vi "AFM_sync_volumetric_scan.vi"() -> ()   [LabVIEW 2017]
uses:
  <vilib>/DAQmx/write.llb/DAQmx Write (Analog DBL 1Chan 1Samp).vi
  <vilib>/DAQmx/write.llb/DAQmx Write (Analog 1D DBL NChan 1Samp).vi
  <vilib>/DAQmx/write.llb/DAQmx Write (Analog 2D DBL NChan NSamp).vi
  <vilib>/Utility/file.llb/Read Delimited Spreadsheet (DBL).vi
  <vilib>/DAQmx/create/channels.llb/DAQmx Create Channel (AO-Voltage-Basic).vi
  <vilib>/DAQmx/miscellaneous.llb/DAQmx Fill In Error Info.vi
  <vilib>/measure/mascope.llb/Transition Measurements 1 chan.vi
  <vilib>/DAQmx/configure/timing.llb/DAQmx Timing (Sample Clock).vi
  <vilib>/DAQmx/configure/trigger.llb/DAQmx Start Trigger (Digital Edge).vi
  <resource>/objmgr/daqmx.rc
  <vilib>/measure/NI_MAPro.lvlib
panel:
  out "Sampling rate":i32
  out "ETL3":waveform(dbl)(graph)
  out "mirror y":waveform(dbl)(graph)
  out "mirror x":waveform(dbl)(graph)
  out "561":waveform(dbl)(graph)
  out "488":waveform(dbl)(graph)
  out "camera":waveform(dbl)(graph)
  out "mirx transition duration":dbl
  out "transition duration":dbl
  out "etl3 timing array":dbl[](array[numeric])
  out "mirror y timing array":dbl[](array[numeric])
  out "mirror x timing array":dbl[](array[numeric])
  out "561 timing array":dbl[](array[numeric])
  out "488 timing array":dbl[](array[numeric])
  out "camera timing array":dbl[](array[numeric])
  out "etl raw":dbl[](array[numeric])
  out "miry raw":dbl[](array[numeric])
  out "mirx raw":dbl[](array[numeric])
  out "561 Intensity":dbl
  out "488 Intensity":dbl
  out "Off Time":dbl
  out "On Time":dbl
  out "Number of slices":dbl
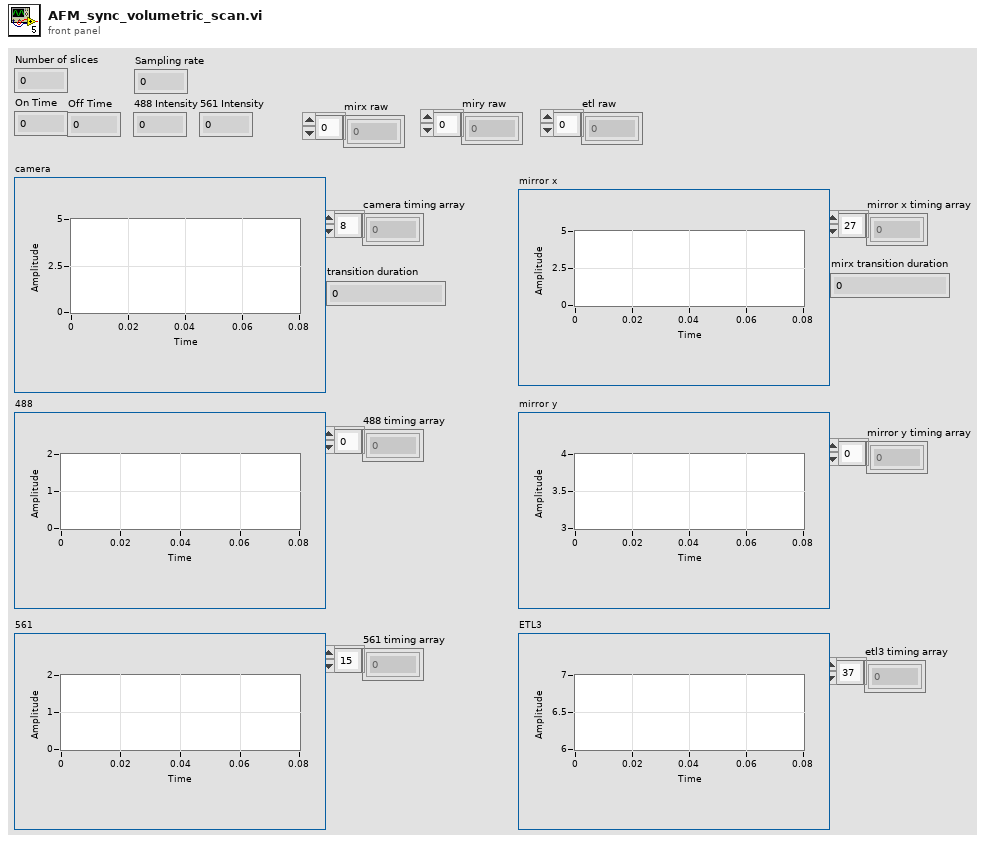
[diagram p1: front panel]
types:
  T1 = enum32{"Invalid", "Standard", "Closed", "Hidden", "Minimized", "Maximized"}
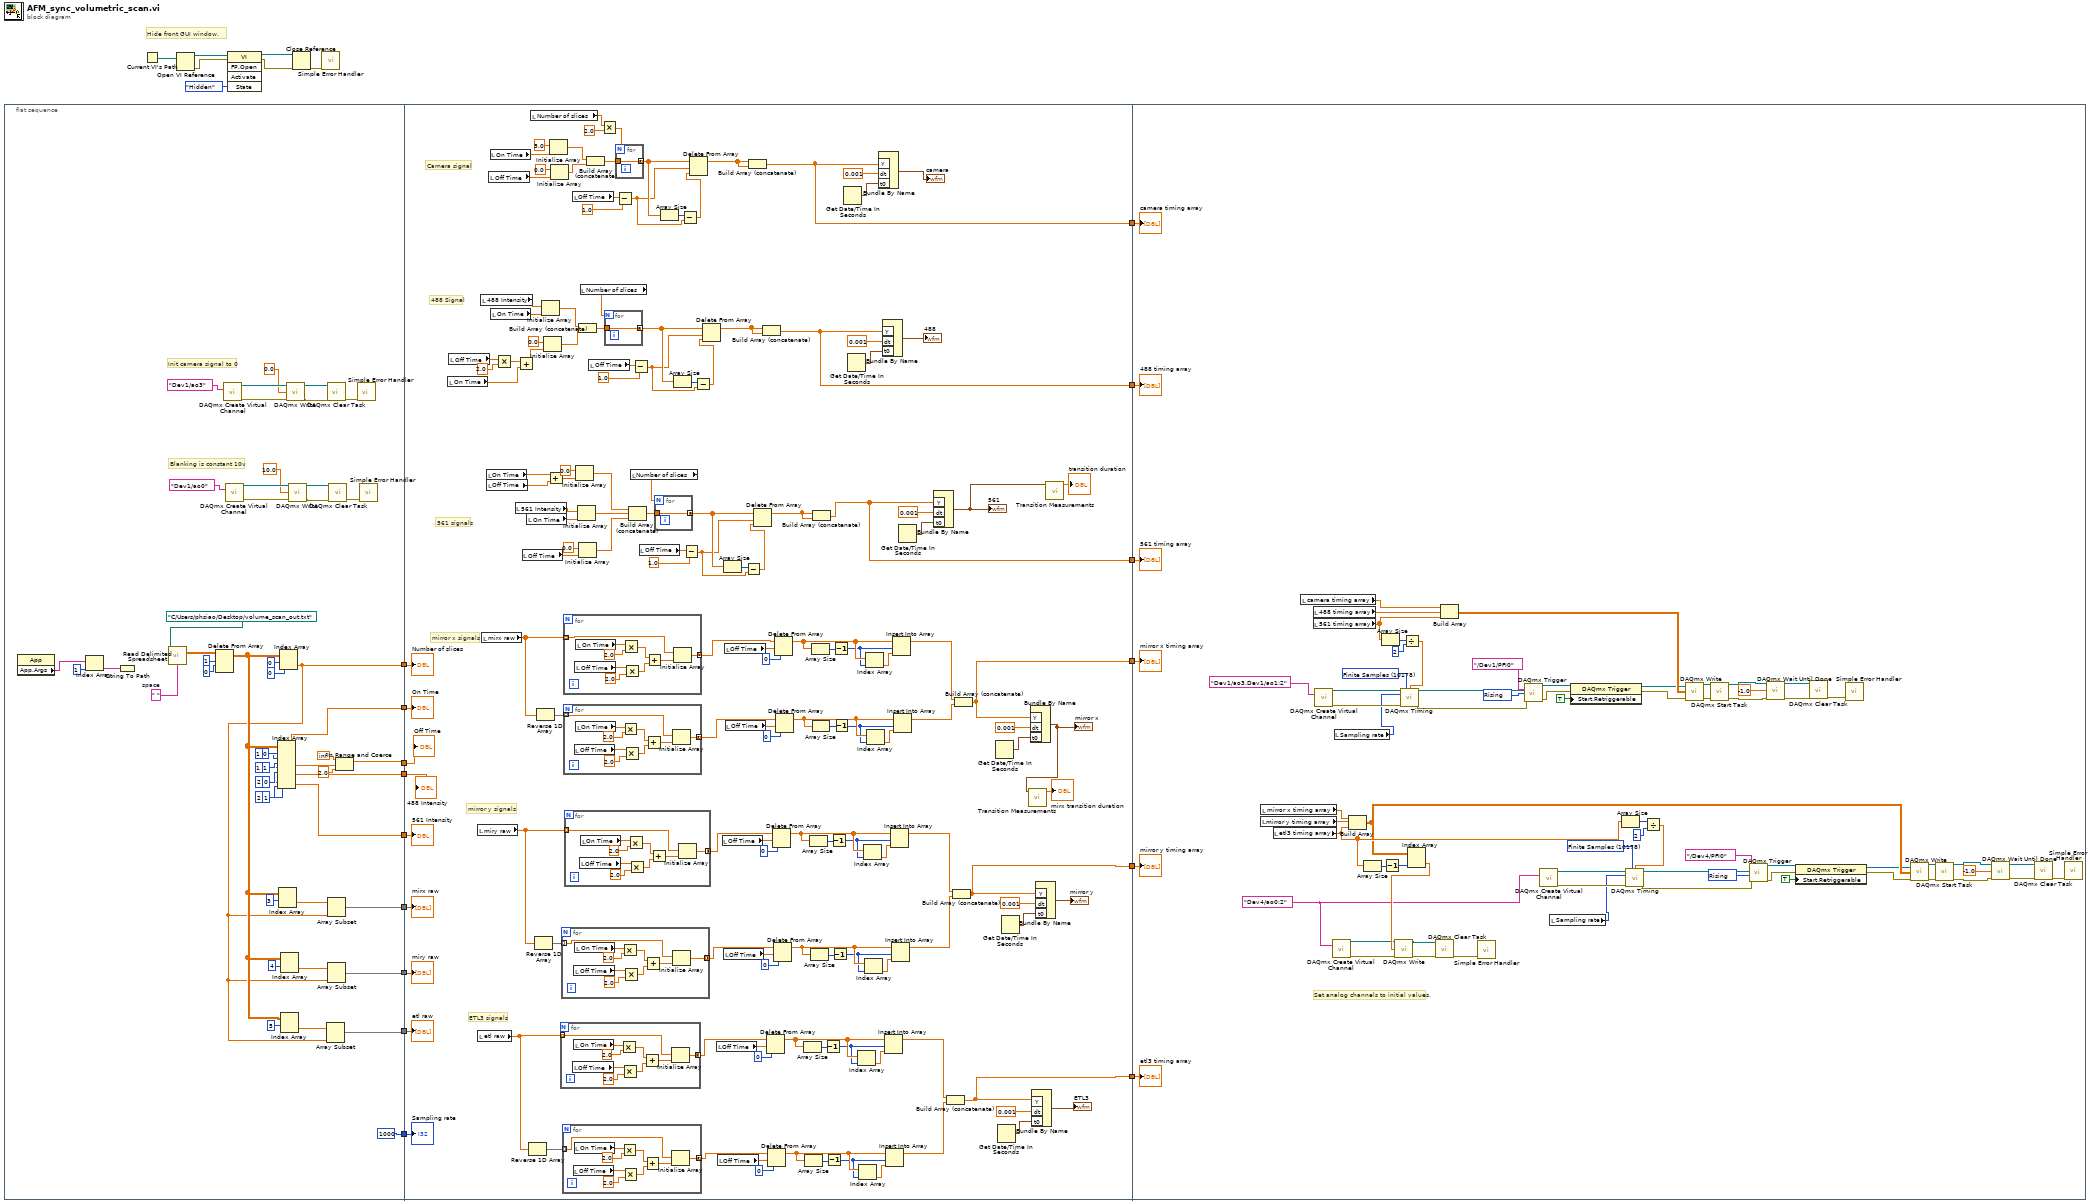
[diagram p0: block diagram]
diagram:
  # "Hide front GUI window."
  n1 = flat-sequence {
    tunnel: [w48] -> w22
    tunnel: [w47] -> w21
    tunnel: [w46] -> w20
    tunnel: [w45] -> w19
    tunnel: [w44] -> w18
    tunnel: [w43] -> w17
    tunnel: [w42] -> w16
    tunnel: [w41] -> w15
    tunnel: [1000] -> w8
    tunnel: w22 -> [w96]
    tunnel: w21 -> [w95]
    tunnel: w20 -> [w94]
    tunnel: w19 -> [w93]
    tunnel: w18 -> [w92]
    tunnel: w17 -> [w91]
    tunnel: w16 -> [w90]
    tunnel: w15 -> [w89]
    tunnel: [w88] -> w14
    tunnel: [w87] -> w13
    tunnel: [w86] -> w12
    tunnel: [w85] -> w11
    tunnel: [w84] -> w10
    tunnel: [w83] -> w9
    tunnel: w8 -> [w74]
    tunnel: w14 -> [w283]
    tunnel: w13 -> [w282]
    tunnel: w12 -> [w281]
    tunnel: w11 -> [w280]
    tunnel: w10 -> [w279]
    tunnel: w9 -> [w278]
    frame #0 {
      w49 = " "  # space
      # "Init camera signal to 0"
      # "Blanking is constant 10v"
      n2 = property class="App"() -> ("App.Args"=w24:string[])  [unwired: 2 in, 2 out]
      n3 = Index Array(array=w24, index=1) -> (element=w23:string)
      n4 = String To Path(string=w23) -> ()  [unwired: 1 out]
      n5 = call-poly <vilib>:"Read Delimited Spreadsheet.vi"("file path (dialog if empty)"=path "C:/Users/phsiao/Desktop/volume_scan_out.txt", "delimiter (\\t)"=w49) -> ("all rows"=w68:dbl[][])  [unwired: 8 in, 5 out]
      n6 = Delete From Array(array=w68, length=1, index (row)=0) -> (array with subset deleted=w69:dbl[][])  [unwired: 1 in, 1 out]
      n7 = call-poly <vilib>:"DAQmx Create Virtual Channel.vi"("physical channels"=tag "Dev1/ao3") -> ("task out"=w29:refnum<k21>, "error out"=w30:errorcluster)  [unwired: 13 in]
      n8 = call-poly <vilib>:"DAQmx Create Virtual Channel.vi"("physical channels"=tag "Dev1/ao0") -> ("task out"=w37:refnum<k21>, "error out"=w38:errorcluster)  [unwired: 13 in]
      n9 = Index Array(array=w69, index (row) #1=1 ("index (row)"), index (col) #1=0 ("disabled index (col)"), index (row) #2=1 ("index (row)"), index (col) #2=1 ("disabled index (col)"), index (row) #3=2 ("index (row)"), index (col) #3=0 ("disabled index (col)"), index (row) #4=2 ("index (row)"), index (col) #4=1 ("disabled index (col)")) -> (element #1=w47:dbl, element #2=w73:dbl, element #3=w45:dbl, element #4=w44:dbl)
      n10 = Index Array(array=w69, index (row)=3) -> (element=w70:dbl[])  [unwired: 1 in]
      n11 = Index Array(array=w69, index (row)=0, index (col)=0 ("disabled index (col)")) -> (element=w48:dbl)
      n12 = Index Array(array=w69, index (row)=5) -> (element=w72:dbl[])  [unwired: 1 in]
      n13 = Index Array(array=w69, index (row)=4) -> (element=w71:dbl[])  [unwired: 1 in]
      n14 = call-poly <vilib>:"DAQmx Write.vi"("task/channels in"=w29, "data"=0.0, "error in"=w30) -> ("task out"=w31:refnum<k21>, "error out"=w32:errorcluster)  [unwired: 10 in, 1 out]
      n15 = call-poly <vilib>:"DAQmx Write.vi"("task/channels in"=w37, "data"=10.0, "error in"=w38) -> ("task out"=w39:refnum<k21>, "error out"=w40:errorcluster)  [unwired: 10 in, 1 out]
      n16 = Array Subset(array=w72, length=w48) -> (w41:dbl[])  [unwired: 1 in]
      n17 = call <vilib>:"DAQmx Clear Task.vi"("task in"=w31, "error in"=w32) -> ("error out"=w28:errorcluster)  [unwired: 13 in]
      n18 = Array Subset(array=w70, length=w48) -> (w43:dbl[])  [unwired: 1 in]
      n19 = Array Subset(array=w71, length=w48) -> (w42:dbl[])  [unwired: 1 in]
      n20 = call <vilib>:"DAQmx Clear Task.vi"("task in"=w39, "error in"=w40) -> ("error out"=w36:errorcluster)  [unwired: 13 in]
      n21 = In Range and Coerce(upper limit=inf, x=w73, lower limit=2.0) -> (coerced(x)=w46:dbl)  [unwired: 1 out]
      n22 = call <vilib>:"Simple Error Handler.vi"("error in (no error)"=w28) -> ()  [unwired: 4 in, 5 out]
      n23 = call <vilib>:"Simple Error Handler.vi"("error in (no error)"=w36) -> ()  [unwired: 4 in, 5 out]
    }
    frame #1 {
      # "ETL3 signals"
      # "mirror y signals"
      # "mirror x signals"
      # "561 signals"
      # "488 Signal"
      # "Camera signal"
      n24 = local read "On Time"() -> (w194:dbl)
      n25 = local read "Off Time"() -> (w197:dbl)
      n26 = local read "miry raw"() -> (w123:dbl[])
      n27 = local read "etl raw"() -> (w119:dbl[])
      n28 = local read "488 Intensity"() -> (w201:dbl)
      n29 = local read "mirx raw"() -> (w127:dbl[])
      n30 = local read "On Time"() -> (w168:dbl)
      n31 = local read "Off Time"() -> (w179:dbl)
      n32 = local read "Off Time"() -> (w216:dbl)
      n33 = local read "On Time"() -> (w217:dbl)
      n34 = local read "On Time"() -> (w200:dbl)
      n35 = Multiply(x=w197, y=2.0) -> (x*y=w195:dbl)
      n36 = local read "561 Intensity"() -> (w182:dbl)
      n37 = Add(x=w195, y=w194) -> (x+y=w193:dbl)
      n38 = local read "Off Time"() -> (w164:dbl)
      n39 = local read "On Time"() -> (w181:dbl)
      n40 = Reverse 1D Array(array=w119) -> (reversed array=w117:dbl[])
      n41 = local read "Number of slices"() -> (w209:dbl)
      n42 = Reverse 1D Array(array=w123) -> (reversed array=w121:dbl[])
      n43 = Reverse 1D Array(array=w127) -> (reversed array=w125:dbl[])
      n44 = Initialize Array(w201, w200) -> (w199:dbl[])
      n45 = Initialize Array(0.0 ("element"), w193) -> (w192:dbl[])
      n46 = Add(x=w168, y=w179) -> (x+y=w178:dbl)
      n47 = Initialize Array(5.0 ("element"), w217) -> (w214:dbl[])
      n48 = Initialize Array(0.0 ("element"), w216) -> (w213:dbl[])
      n49 = for {
        tunnel: w119 -> [w229] mode=indexing
        tunnel: [w228] -> w118 mode=concatenating
        n50 = local read "Off Time"() -> (w234:dbl)
        n51 = local read "On Time"() -> (w232:dbl)
        n52 = Multiply(x=w232, y=2.0) -> (x*y=w233:dbl)
        n53 = Multiply(x=w234, y=2.0) -> (x*y=w235:dbl)
        n54 = Add(x=w233, y=w235) -> (x+y=w236:dbl)
        n55 = Initialize Array(w229, w236) -> (w228:dbl[])
      }
      n56 = for {
        tunnel: w121 -> [w238] mode=indexing
        tunnel: [w237] -> w120 mode=concatenating
        n57 = local read "Off Time"() -> (w243:dbl)
        n58 = local read "On Time"() -> (w241:dbl)
        n59 = Multiply(x=w241, y=2.0) -> (x*y=w242:dbl)
        n60 = Multiply(x=w243, y=2.0) -> (x*y=w244:dbl)
        n61 = Add(x=w242, y=w244) -> (x+y=w245:dbl)
        n62 = Initialize Array(w238, w245) -> (w237:dbl[])
      }
      n63 = for {
        tunnel: w117 -> [w220] mode=indexing
        tunnel: [w219] -> w116 mode=concatenating
        n64 = local read "Off Time"() -> (w225:dbl)
        n65 = local read "On Time"() -> (w223:dbl)
        n66 = Multiply(x=w223, y=2.0) -> (x*y=w224:dbl)
        n67 = Multiply(x=w225, y=2.0) -> (x*y=w226:dbl)
        n68 = Add(x=w224, y=w226) -> (x+y=w227:dbl)
        n69 = Initialize Array(w220, w227) -> (w219:dbl[])
      }
      n70 = for {
        tunnel: w127 -> [w265] mode=indexing
        tunnel: [w264] -> w126 mode=concatenating
        n71 = local read "Off Time"() -> (w270:dbl)
        n72 = local read "On Time"() -> (w272:dbl)
        n73 = Multiply(x=w272, y=2.0) -> (x*y=w271:dbl)
        n74 = Multiply(x=w270, y=2.0) -> (x*y=w269:dbl)
        n75 = Add(x=w271, y=w269) -> (x+y=w268:dbl)
        n76 = Initialize Array(w265, w268) -> (w264:dbl[])
      }
      n77 = for {
        tunnel: w125 -> [w256] mode=indexing
        tunnel: [w255] -> w124 mode=concatenating
        n78 = local read "Off Time"() -> (w261:dbl)
        n79 = local read "On Time"() -> (w263:dbl)
        n80 = Multiply(x=w263, y=2.0) -> (x*y=w262:dbl)
        n81 = Multiply(x=w261, y=2.0) -> (x*y=w260:dbl)
        n82 = Add(x=w262, y=w260) -> (x+y=w259:dbl)
        n83 = Initialize Array(w256, w259) -> (w255:dbl[])
      }
      n84 = for {
        tunnel: w123 -> [w247] mode=indexing
        tunnel: [w246] -> w122 mode=concatenating
        n85 = local read "Off Time"() -> (w252:dbl)
        n86 = local read "On Time"() -> (w250:dbl)
        n87 = Multiply(x=w250, y=2.0) -> (x*y=w251:dbl)
        n88 = Multiply(x=w252, y=2.0) -> (x*y=w253:dbl)
        n89 = Add(x=w251, y=w253) -> (x+y=w254:dbl)
        n90 = Initialize Array(w247, w254) -> (w246:dbl[])
      }
      n91 = local read "Off Time"() -> (w208:dbl)
      n92 = Initialize Array(0.0 ("element"), w178) -> (w167:dbl[])
      n93 = Initialize Array(w182, w181) -> (w166:dbl[])
      n94 = Initialize Array(0.0 ("element"), w164) -> (w163:dbl[])
      n95 = Build Array (concatenate)(w199, w192) -> (w190:dbl[])
      n96 = local read "Number of slices"() -> (w191:dbl)
      n97 = Build Array (concatenate)(w214, w213) -> (w212:dbl[])
      n98 = local read "Off Time"() -> (w186:dbl)
      n99 = Multiply(x=w209, y=2.0) -> (x*y=w211:dbl)
      n100 = for {
        N: w191 -> [_]
        tunnel: w190 -> [w274]
        tunnel: [w274] -> w187 mode=concatenating
      }
      n101 = for {
        N: w211 -> [_]
        tunnel: w212 -> [w275]
        tunnel: [w275] -> w206 mode=concatenating
      }
      n102 = Subtract(x=w208, y=1.0) -> (x-y=w204:dbl)
      n103 = Build Array (concatenate)(w167, w166, w163) -> (w176:dbl[])
      n104 = local read "Number of slices"() -> (w177:dbl)
      n105 = Subtract(x=w186, y=1.0) -> (x-y=w184:dbl)
      n106 = local read "Off Time"() -> (w172:dbl)
      n107 = for {
        N: w177 -> [_]
        tunnel: w176 -> [w273]
        tunnel: [w273] -> w173 mode=concatenating
      }
      n108 = Array Size(array=w206) -> (size(s)=w205:i32)
      n109 = Array Size(array=w187) -> (size(s)=w189:i32)
      n110 = Subtract(x=w205, y=w204) -> (x-y=w203:dbl)
      n111 = Subtract(x=w172, y=1.0) -> (x-y=w170:dbl)
      n112 = Delete From Array(array=w206, length=w204, index=w203) -> (array with subset deleted=w202:dbl[])  [unwired: 1 out]
      n113 = Subtract(x=w189, y=w184) -> (x-y=w188:dbl)
      n114 = Delete From Array(array=w187, length=w184, index=w188) -> (array with subset deleted=w183:dbl[])  [unwired: 1 out]
      n115 = local read "Off Time"() -> (w138:dbl)
      n116 = local read "Off Time"() -> (w133:dbl)
      n117 = local read "Off Time"() -> (w150:dbl)
      n118 = local read "Off Time"() -> (w145:dbl)
      n119 = Array Size(array=w173) -> (size(s)=w175:i32)
      n120 = local read "Off Time"() -> (w162:dbl)
      n121 = local read "Off Time"() -> (w157:dbl)
      n122 = Subtract(x=w175, y=w170) -> (x-y=w174:dbl)
      n123 = Build Array (concatenate)(w202, w202) -> (w88:dbl[])
      n124 = Delete From Array(array=w173, length=w170, index=w174) -> (array with subset deleted=w169:dbl[])  [unwired: 1 out]
      n125 = Build Array (concatenate)(w183, w183) -> (w87:dbl[])
      n126 = Delete From Array(array=w118, length=w138, index=0) -> (array with subset deleted=w135:dbl[])  [unwired: 1 out]
      n127 = Delete From Array(array=w116, length=w133, index=0) -> (array with subset deleted=w130:dbl[])  [unwired: 1 out]
      n128 = Delete From Array(array=w122, length=w150, index=0) -> (array with subset deleted=w147:dbl[])  [unwired: 1 out]
      n129 = Delete From Array(array=w120, length=w145, index=0) -> (array with subset deleted=w142:dbl[])  [unwired: 1 out]
      n130 = Delete From Array(array=w126, length=w162, index=0) -> (array with subset deleted=w159:dbl[])  [unwired: 1 out]
      n131 = Delete From Array(array=w124, length=w157, index=0) -> (array with subset deleted=w154:dbl[])  [unwired: 1 out]
      n132 = Array Size(array=w135) -> (size(s)=w137:i32)
      n133 = Array Size(array=w130) -> (size(s)=w132:i32)
      n134 = Array Size(array=w147) -> (size(s)=w149:i32)
      n135 = Array Size(array=w142) -> (size(s)=w144:i32)
      n136 = Array Size(array=w159) -> (size(s)=w161:i32)
      n137 = Array Size(array=w154) -> (size(s)=w156:i32)
      n138 = Build Array (concatenate)(w169, w169) -> (w86:dbl[])
      n139 = Decrement(x=w137) -> (x-1=w134:i32)
      n140 = Decrement(x=w132) -> (x-1=w129:i32)
      n141 = Decrement(x=w149) -> (x-1=w146:i32)
      n142 = Decrement(x=w144) -> (x-1=w141:i32)
      n143 = Decrement(x=w161) -> (x-1=w158:i32)
      n144 = Decrement(x=w156) -> (x-1=w153:i32)
      n145 = Get Date/Time In Seconds() -> (seconds since 1Jan1904=w110:timestamp)
      n146 = Get Date/Time In Seconds() -> (seconds since 1Jan1904=w108:timestamp)
      n147 = Index Array(array=w135, index=w134) -> (element=w136:dbl)
      n148 = Index Array(array=w130, index=w129) -> (element=w131:dbl)
      n149 = Index Array(array=w147, index=w146) -> (element=w148:dbl)
      n150 = Index Array(array=w142, index=w141) -> (element=w143:dbl)
      n151 = Index Array(array=w159, index=w158) -> (element=w160:dbl)
      n152 = Index Array(array=w154, index=w153) -> (element=w155:dbl)
      n153 = Bundle By Name("Y"=w88, "dt"=0.001, "t0"=w110) -> (→"camera":waveform(dbl))  [unwired: 1 in]
      n154 = Bundle By Name("Y"=w87, "dt"=0.001, "t0"=w108) -> (→"488":waveform(dbl))  [unwired: 1 in]
      n155 = Insert Into Array(array=w135, index=w134, new element=w136) -> (w128:dbl[])
      n156 = Insert Into Array(array=w130, index=w129, new element=w131) -> (w103:dbl[])
      n157 = Insert Into Array(array=w147, index=w146, new element=w148) -> (w140:dbl[])
      n158 = Insert Into Array(array=w142, index=w141, new element=w143) -> (w139:dbl[])
      n159 = Insert Into Array(array=w159, index=w158, new element=w160) -> (w152:dbl[])
      n160 = Insert Into Array(array=w154, index=w153, new element=w155) -> (w151:dbl[])
      n161 = Get Date/Time In Seconds() -> (seconds since 1Jan1904=w112:timestamp)
      n162 = Bundle By Name("Y"=w86, "dt"=0.001, "t0"=w112) -> (w78:waveform(dbl))  [unwired: 1 in]
      "561" <- w78
      n163 = Build Array (concatenate)(w128, w103) -> (w83:dbl[])
      n164 = Build Array (concatenate)(w140, w139) -> (w84:dbl[])
      n165 = Build Array (concatenate)(w152, w151) -> (w85:dbl[])
      n166 = Get Date/Time In Seconds() -> (seconds since 1Jan1904=w114:timestamp)
      n167 = Get Date/Time In Seconds() -> (seconds since 1Jan1904=w104:timestamp)
      n168 = Get Date/Time In Seconds() -> (seconds since 1Jan1904=w106:timestamp)
      n169 = Bundle By Name("Y"=w85, "dt"=0.001, "t0"=w114) -> (w77:waveform(dbl))  [unwired: 1 in]
      "mirror x" <- w77
      n170 = call-poly <vilib>:"Transition Measurements.vi"("signal in"=w77) -> ("transition duration"=→"mirx transition duration":dbl)  [unwired: 5 in, 5 out]
      n171 = Bundle By Name("Y"=w83, "dt"=0.001, "t0"=w104) -> (→"ETL3":waveform(dbl))  [unwired: 1 in]
      n172 = Bundle By Name("Y"=w84, "dt"=0.001, "t0"=w106) -> (→"mirror y":waveform(dbl))  [unwired: 1 in]
      n173 = call-poly <vilib>:"Transition Measurements.vi"("signal in"=w78) -> ("transition duration"=→"transition duration":dbl)  [unwired: 5 in, 5 out]
      "Number of slices" <- w96
      "On Time" <- w95
      "Off Time" <- w94
      "488 Intensity" <- w93
      "561 Intensity" <- w92
      "mirx raw" <- w91
      "miry raw" <- w90
      "etl raw" <- w89
      "Sampling rate" <- w74
    }
    frame #2 {
      w294 = 10280 items=["Rising"=10280, "Falling"=10171] ("edge")
      w291 = 10178 items=["Finite Samples"=10178, "Continuous Samples"=10123, "Hardware Timed Single Point"=12522] ("sample mode")
      w293 = tag "Dev4/ao0:2" ("physical channels")
      w287 = 10280 items=["Rising"=10280, "Falling"=10171] ("edge")
      w284 = 10178 items=["Finite Samples"=10178, "Continuous Samples"=10123, "Hardware Timed Single Point"=12522] ("sample mode")
      # "Set analog channels to initial values."
      n174 = local read "mirror y timing array"() -> (w320:dbl[])
      n175 = local read "mirror x timing array"() -> (w321:dbl[])
      n176 = local read "etl3 timing array"() -> (w346:dbl[])
      n177 = local read "camera timing array"() -> (w318:dbl[])
      n178 = local read "488 timing array"() -> (w317:dbl[])
      n179 = local read "561 timing array"() -> (w323:dbl[])
      n180 = call-poly <vilib>:"DAQmx Create Virtual Channel.vi"("physical channels"=tag "Dev1/ao3,Dev1/ao1:2") -> ("task out"=w305:refnum<k21>, "error out"=w306:errorcluster)  [unwired: 13 in]
      n181 = call-poly <vilib>:"DAQmx Create Virtual Channel.vi"("physical channels"=w293) -> ("task out"=w313:refnum<k21>, "error out"=w314:errorcluster)  [unwired: 13 in]
      n182 = local read "Sampling rate"() -> (w277:i32)
      n183 = Build Array(w321, w320, w346) -> (w345:dbl[][])
      n184 = Array Size(array=w346) -> (size(s)=w325:i32)
      n185 = Array Size(array=w323) -> (size(s)=w322:i32)
      n186 = Decrement(x=w325) -> (x-1=w326:i32)
      n187 = Divide(x=w322, y=2) -> (x/y=w324:dbl)
      n188 = call-poly <vilib>:"DAQmx Timing.vi"("task/channels in"=w305, "sample mode"=w284, "samples per channel"=w324, "rate"=w277, "error in"=w306) -> ("task out"=w307:refnum<k21>, "error out"=w308:errorcluster)  [unwired: 9 in]
      n189 = Index Array(array=w345, index (col)=w326) -> (element=w327:dbl[])  [unwired: 1 in]
      n190 = call-poly <vilib>:"DAQmx Write.vi"("task/channels in"=w313, "data"=w327, "error in"=w314) -> ("task out"=w315:refnum<k21>, "error out"=w316:errorcluster)  [unwired: 10 in, 1 out]
      n191 = call <vilib>:"DAQmx Clear Task.vi"("task in"=w315, "error in"=w316) -> ("error out"=w347:errorcluster)  [unwired: 13 in]
      n192 = Build Array(w318, w317, w323) -> (w319:dbl[][])
      n193 = call <vilib>:"Simple Error Handler.vi"("error in (no error)"=w347) -> ()  [unwired: 4 in, 5 out]
      n194 = call-poly <vilib>:"DAQmx Trigger.vi"("task/channels in"=w307, "source"=tag "/Dev1/PFI0", "edge"=w287, "error in"=w308) -> ("task out"=w309:refnum<k21>, "error out"=w312:errorcluster)  [unwired: 10 in]
      n195 = call-poly <vilib>:"DAQmx Create Virtual Channel.vi"("physical channels"=w293) -> ("task out"=w335:refnum<k21>, "error out"=w336:errorcluster)  [unwired: 13 in]
      n196 = local read "Sampling rate"() -> (w276:i32)
      n197 = property class="DAQmx Trigger"(reference=w309, error in=w312, "Start.Retriggerable"=TRUE) -> (reference out=w310:refnum<k21>, error out=w311:errorcluster)
      n198 = Array Size(array=w346) -> (size(s)=w343:i32)
      n199 = Divide(x=w343, y=2) -> (x/y=w344:dbl)
      n200 = call-poly <vilib>:"DAQmx Timing.vi"("task/channels in"=w335, "sample mode"=w291, "samples per channel"=w344, "rate"=w276, "error in"=w336) -> ("task out"=w337:refnum<k21>, "error out"=w338:errorcluster)  [unwired: 9 in]
      n201 = call-poly <vilib>:"DAQmx Write.vi"("task/channels in"=w310, "data"=w319, "error in"=w311) -> ("task out"=w303:refnum<k21>, "error out"=w304:errorcluster)  [unwired: 10 in, 1 out]
      n202 = call <vilib>:"DAQmx Start Task.vi"("task/channels in"=w303, "error in"=w304) -> ("task out"=w302:refnum<k21>, "error out"=w301:errorcluster)  [unwired: 12 in]
      n203 = call-poly <vilib>:"DAQmx Trigger.vi"("task/channels in"=w337, "source"=tag "/Dev4/PFI0", "edge"=w294, "error in"=w338) -> ("task out"=w339:refnum<k21>, "error out"=w342:errorcluster)  [unwired: 10 in]
      n204 = call <vilib>:"DAQmx Wait Until Done.vi"("task/channels in"=w302, "timeout (sec)"=-1.0, "error in"=w301) -> ("task out"=w299:refnum<k21>, "error out"=w300:errorcluster)  [unwired: 11 in]
      n205 = property class="DAQmx Trigger"(reference=w339, error in=w342, "Start.Retriggerable"=TRUE) -> (reference out=w340:refnum<k21>, error out=w341:errorcluster)
      n206 = call <vilib>:"DAQmx Clear Task.vi"("task in"=w299, "error in"=w300) -> ("error out"=w298:errorcluster)  [unwired: 13 in]
      n207 = call <vilib>:"Simple Error Handler.vi"("error in (no error)"=w298) -> ()  [unwired: 4 in, 5 out]
      n208 = call-poly <vilib>:"DAQmx Write.vi"("task/channels in"=w340, "data"=w345, "error in"=w341) -> ("task out"=w333:refnum<k21>, "error out"=w334:errorcluster)  [unwired: 10 in, 1 out]
      n209 = call <vilib>:"DAQmx Start Task.vi"("task/channels in"=w333, "error in"=w334) -> ("task out"=w332:refnum<k21>, "error out"=w331:errorcluster)  [unwired: 12 in]
      n210 = call <vilib>:"DAQmx Wait Until Done.vi"("task/channels in"=w332, "timeout (sec)"=-1.0, "error in"=w331) -> ("task out"=w329:refnum<k21>, "error out"=w330:errorcluster)  [unwired: 11 in]
      n211 = call <vilib>:"DAQmx Clear Task.vi"("task in"=w329, "error in"=w330) -> ("error out"=w328:errorcluster)  [unwired: 13 in]
      n212 = call <vilib>:"Simple Error Handler.vi"("error in (no error)"=w328) -> ()  [unwired: 4 in, 5 out]
      "camera timing array" <- w283
      "488 timing array" <- w282
      "561 timing array" <- w281
      "mirror x timing array" <- w280
      "mirror y timing array" <- w279
      "etl3 timing array" <- w278
    }
  }
  n213 = Current VI's Path() -> (path=w7:path)
  n214 = Open VI Reference(vi path=w7) -> (vi reference=w5:refnum<vi>, error out=w4:errorcluster)  [unwired: 5 in]
  n215 = invoke class="VI" method="FP.Open"(reference=w5, error in=w4, "State"=T1."Hidden") -> (reference out=w3:refnum<vi>, error out=w2:errorcluster)  [unwired: 2 in, 3 out]
  n216 = Close Reference(reference=w3, error in (no error)=w2) -> (error out=w6:errorcluster)
  n217 = call <vilib>:"Simple Error Handler.vi"("error in (no error)"=w6) -> ()  [unwired: 4 in, 5 out]
